vi "5-3 all about typedefs.vi"() -> ()   [LabVIEW 2015]
uses:
  stricttype def numeric.ctl
  type def numeric.ctl
panel:
  in  "Type Def Numeric 2":dbl
  in  "Type Def Numeric":T1
  in  "Strict Type def numeric":T2
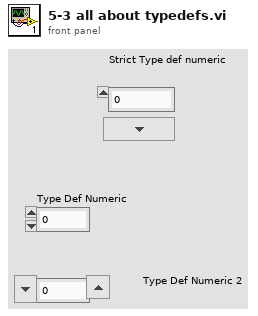
[diagram p1: front panel]
types:
  T1 = typedef "type def numeric.ctl" = dbl
  T2 = typedef "stricttype def numeric.ctl" = dbl
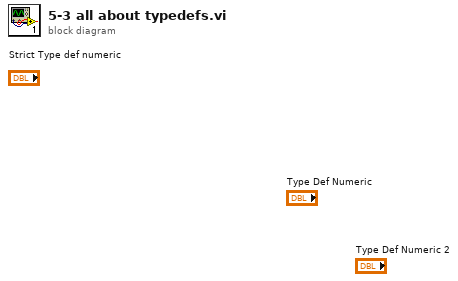
[diagram p0: block diagram]
diagram:
